vi "Ping Response.vi"(8 "error in (no error)":errorcluster, 9 "Seconds to Respond":dbl, 10 "Actor Core ID":string, 11 "Actor Monitor in":refnum<class "Actor Monitor.lvclass">) -> (0 "error out":errorcluster, 3 "Actor Monitor out":refnum<class "Actor Monitor.lvclass">)   [LabVIEW 2018, in "Monitored Actor.lvlib" / "Actor Monitor.lvclass"]
doc: "Updates the tree to show how long it took to poll the Actor.\n\nCopyright: MGI\nAuthored by: Derek Trepanier"
uses:
  Actor Monitor.lvclass
  UI Info.ctl
  Actor Monitor.lvclass/Actor Monitor.ctl
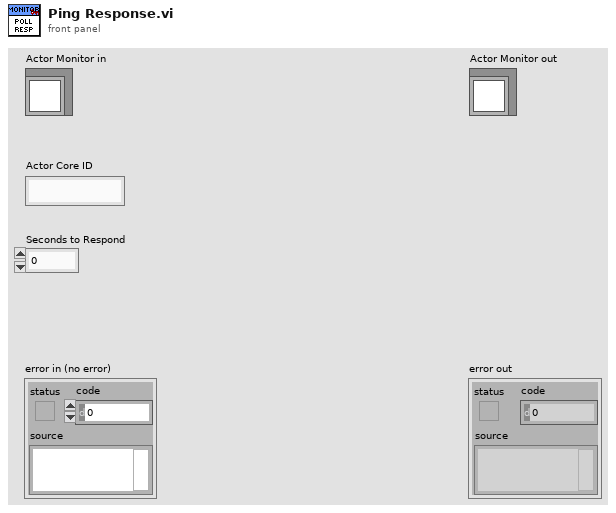
[diagram p1: front panel]
types:
  T1 = typedef "Monitored Actor.lvlib/Actor Monitor.lvclass/UI Info.ctl" = cluster{"Class Name":string, "Actor Core Name":string, "Ping Response Str":string}
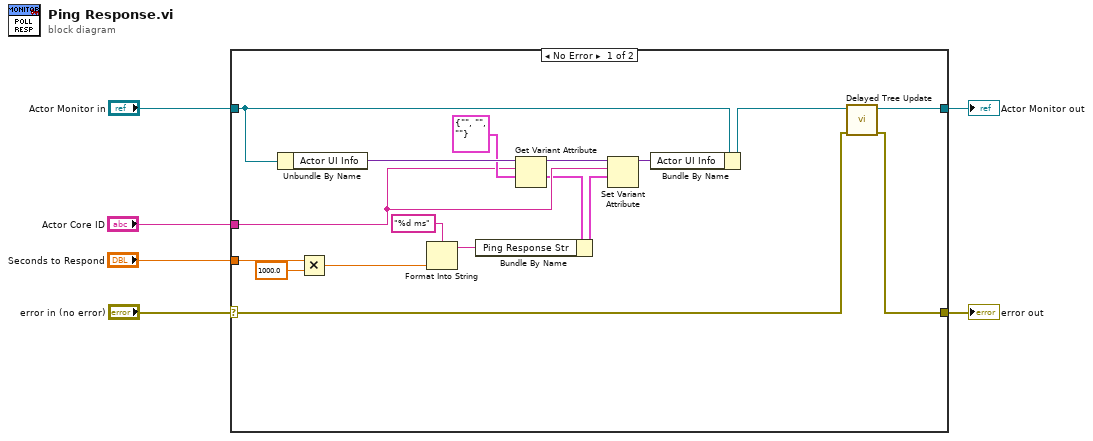
[diagram p0: block diagram]
diagram:
  n1 = case shown="No Error" "error in (no error)" {
    selector: "error in (no error)" -> [w8 w25]
    tunnel: [w7 w25] -> w5
    tunnel: [w9 w24] -> w3
    tunnel: "Actor Monitor in" -> [w23 w24]
    tunnel: "Actor Core ID" -> [w15 _]
    tunnel: "Seconds to Respond" -> [w22 _]
    frame No Error {
      n2 = Unbundle By Name(w23) -> ("Actor UI Info"=w17:variant)
      n3 = Multiply(x=w22, y=1000.0) -> (x*y=w20:dbl)
      n4 = Format Into String(format string="%d ms", w20) -> (resulting string=w12:string)  [unwired: 2 in, 1 out]
      n5 = Get Variant Attribute(Variant=w17, name=w15, default value (empty Variant)=T1 {"Class Name"="", "Actor Core Name"="", "Ping Response Str"=""} ("UI Info")) -> (duplicate Variant=w18:variant, value=w14:T1)  [unwired: 1 in, 2 out]
      n6 = Bundle By Name(cluster=w14, "Ping Response Str"=w12) -> (w13:T1)
      n7 = Set Variant Attribute(Variant=w18, name=w15, value=w13) -> (Variant out=w11:variant)  [unwired: 1 in, 2 out]
      n8 = Bundle By Name(cluster=w23, "Actor UI Info"=w11) -> (w10:refnum<class "Actor Monitor.lvclass">)
      n9 = call "Delayed Tree Update.vi"("error in (no error)"=w8, "Actor Monitor in"=w10) -> ("error out"=w7:errorcluster, "Actor Monitor out"=w9:refnum<class "Actor Monitor.lvclass">)  [unwired: 8 in]
    }
    frame Error {
    }
  }
  "error out" <- w5
  "Actor Monitor out" <- w3
